vi "Display Colour Animation.vi"(8 "error in (no error)":errorcluster, 10 "Animations":T1, 11 "Grove 2 RGB LED Matrix In":refnum<class "Grove 2 RGB LED Matrix.lvclass">) -> (0 "error out":errorcluster, 3 "Grove 2 RGB LED Matrix Out":refnum<class "Grove 2 RGB LED Matrix.lvclass">)   [LabVIEW 2020, in "CTI-Peripheral.lvlib" / "Grove 2 RGB LED Matrix.lvclass"]
uses:
  Grove 2 RGB LED Matrix.lvclass
  Data Types/Animations.ctl
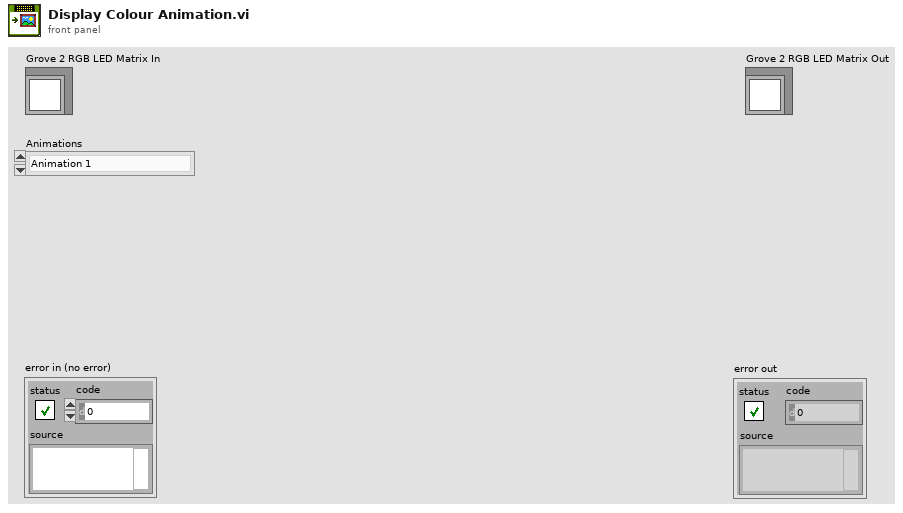
[diagram p1: front panel]
types:
  T1 = typedef "CTI-Peripheral.lvlib/Grove 2 RGB LED Matrix.lvclass/Animations.ctl" = enum16{"Animation 1", "Animation 2", "Rainbow Cycle", "Fire", "Walking", "Broken Heart"}
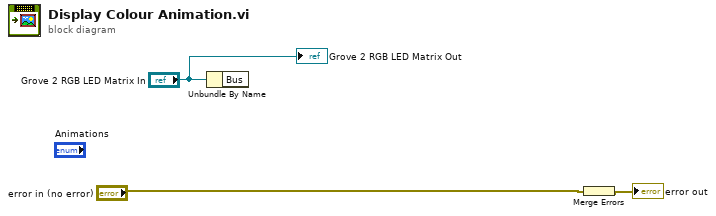
[diagram p0: block diagram]
diagram:
  n1 = Unbundle By Name("Grove 2 RGB LED Matrix In") -> ()  [unwired: 1 out]
  n2 = Merge Errors("error in (no error)") -> (→"error out":errorcluster)
  "Grove 2 RGB LED Matrix Out" <- "Grove 2 RGB LED Matrix In"
